vi "Test Publisher.vi"() -> ()   [LabVIEW 2021]
uses:
  CIFChannels/Typedef/Direction.ctl
  ChannelCommon/typedef/FIFO Config.ctl
  CIF_NIChn_FIFO_DAQ_DVR.lvclass
  ChannelCommon/typedef/TimeStamps.ctl
  ChannelCommon/typedef/Datatype Waveform.ctl
  <vilib>/CIF Foundation/CIF Utilities/DataTypes/Flatten U64.vi
  ChannelCommon/ChannelCommon.lvlib
  CIFChannels/CIFChannels.lvclass
panel:
  in  "stop":bool
  out "timed out?":bool
  out "error out":errorcluster
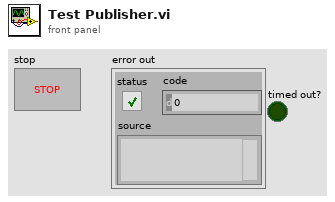
[diagram p1: front panel]
types:
  T1 = typedef "ChannelCommon.lvlib/FIFO Config.ctl" = cluster{"Max Bytes/Msg":u64, "Max Msg/FIFO":u64, "Flags":u64}
  T2 = typedef "CIFChannels.lvclass/Direction.ctl" = enum16{"Publisher", "Subscriber"}
  T3 = typedef "ChannelCommon.lvlib/Datatype Waveform.ctl" = cluster{"measurement":dbl[], "dT":dbl, "Timestamp":i64, "Read Lock":bool}
  T4 = typedef "ChannelCommon.lvlib/TimeStamps.ctl" = cluster{"ClockID":u8, "T0":i64, "T_Out":i64}
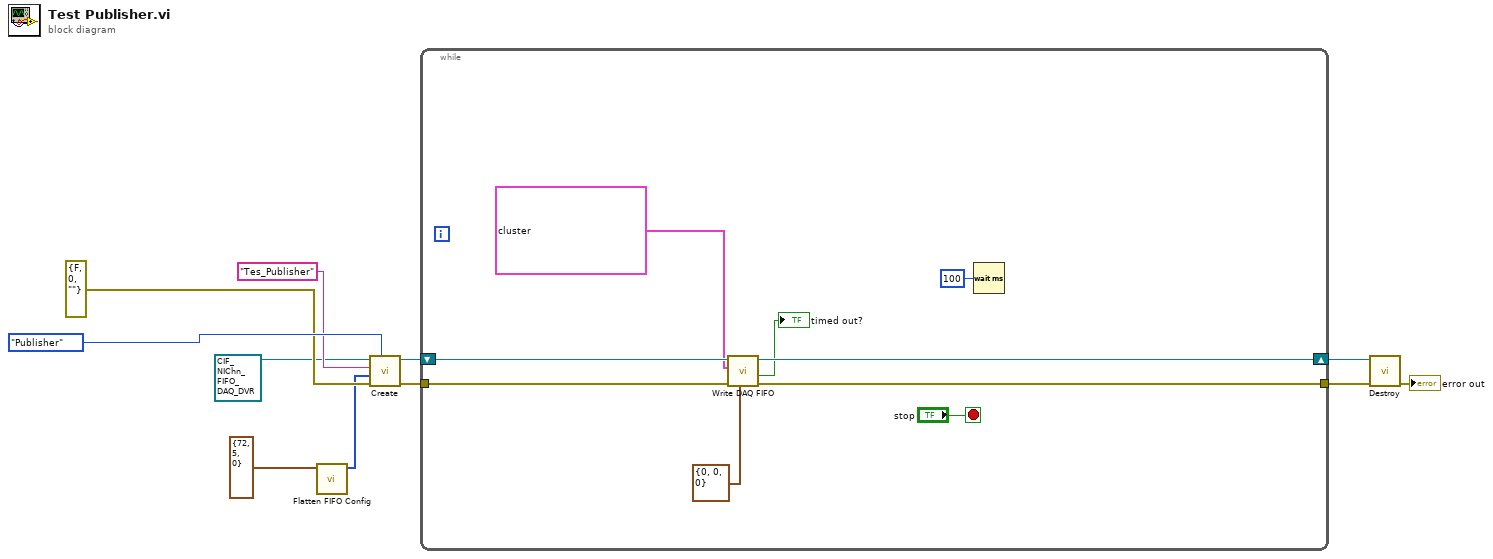
[diagram p0: block diagram]
diagram:
  n1 = call "Flatten FIFO Config.vi"("FIFO Config in"=T1 {"Max Bytes/Msg"=72, "Max Msg/FIFO"=5, "Flags"=0}) -> ("Flattened FIFO Config"=w2:u8[])  [unwired: 10 in]
  n2 = call-dynamic "Create.vi"("Direction"=Direction."Publisher", "error in (no error)"=errorcluster {"status"=FALSE, "code"=0, "source"=""} ("error out"), "Custom Config Data"=w2, "Name"="Tes_Publisher", "CIF_NIChn_FIFO_DAQ in"=refnum<class "CIF_NIChn_FIFO_DAQ_DVR.lvclass"> refnum ("CIF_NIChn_FIFO_DAQ.lvclass")) -> ("error out"=w6:errorcluster, "CIF_NIChn_FIFO_DAQ out"=w7:refnum<class "CIF_NIChn_FIFO_DAQ_DVR.lvclass">)  [unwired: 5 in]
  n3 = while {
    shift-right: [w17] -> w5
    shift-left: w7 -> [w19]
    tunnel: w6 -> [w18]
    tunnel: [w16] -> w4
    stop <- "stop" stop-if-true
    n4 = call-dynamic "Write DAQ FIFO.vi"("FIFO Timestamps"=T4 {"ClockID"=0, "T0"=0, "T_Out"=0}, "error in (no error)"=w18, "Data In"=T3[] [{"measurement"=array[986 elements], "dT"=43.0, "Timestamp"=2, "Read Lock"=FALSE}, {"measurement"=array[1001 elements], "dT"=34.0, "Timestamp"=1, "Read Lock"=FALSE}, {"measurement"=[], "dT"=0.0, "Timestamp"=0, "Read Lock"=FALSE}, {"measurement"=[], "dT"=0.0, "Timestamp"=0, "Read Lock"=FALSE}, {"measurement"=[], "dT"=0.0, "Timestamp"=0, "Read Lock"=FALSE}, {"measurement"=[], "dT"=0.0, "Timestamp"=0, "Read Lock"=FALSE}, {"measurement"=[], "dT"=0.0, "Timestamp"=0, "Read Lock"=FALSE}, {"measurement"=[], "dT"=0.0, "Timestamp"=0, "Read Lock"=FALSE}, {"measurement"=array[100001 elements], "dT"=0.0, "Timestamp"=0, "Read Lock"=FALSE}] ("DAQ In"), "CIF_NIChn_FIFO_DAQ in"=w19) -> ("error out"=w16:errorcluster, "timed out?"=→"timed out?":bool, "CIF_NIChn_FIFO_DAQ out"=w17:refnum<class "CIF_NIChn_FIFO_DAQ_DVR.lvclass">)  [unwired: 4 in, 1 out]
    n5 = Wait (ms)(milliseconds to wait=u32 100) -> ()  [unwired: 1 out]
  }
  n6 = call-dynamic "Destroy.vi"("error in (no error)"=w4, "CIF_NIChn_FIFO_DAQ in"=w5) -> ("error out"=→"error out":errorcluster)  [unwired: 8 in, 1 out]
